vi "normalise_angle.vi"(10 "target -180 .. 180":dbl, 11 "current":dbl) -> (3 "travel_direction":dbl)   [LabVIEW 2017]
uses:
  <vilib>/Analysis/coordinate.llb/Angle Units.ctl
  <vilib>/Analysis/coordinate.llb/Absolute Angle Difference (scalar).vi
  <vilib>/Analysis/coordinate.llb/Wrap Angle (scalar).vi
  <vilib>/Analysis/coordinate.llb/Set Angle Unit.vi
  <vilib>/Analysis/NI_AAL_Angle.lvlib
panel:
  out "s? t:f":dbl
  out "absolute angle difference 2":dbl
  out "absolute angle difference":dbl
  out "current angle (-180..180)":dbl
  out "revolutions":dbl
  out "current angle (0... 359)":dbl
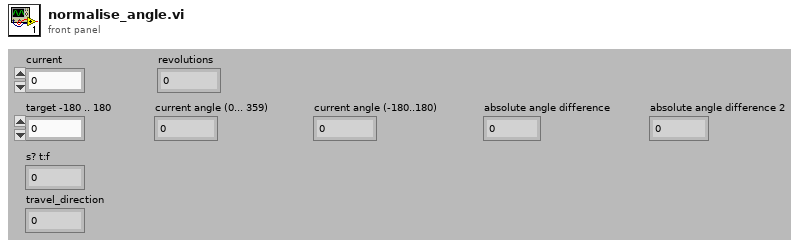
[diagram p1: front panel]
types:
  T1 = typedef "NI_AAL_Angle.lvlib/Angle Units.ctl" = i32
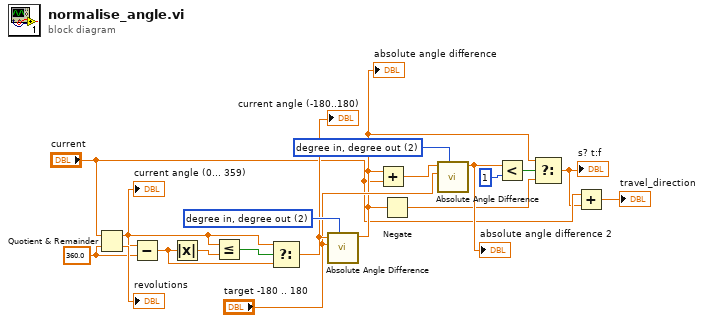
[diagram p0: block diagram]
diagram:
  w10 = T1 2 items=["radian in, radian out", "radian in, degree out", "degree in, degree out", "degree in, radian out"] ("angle units")
  w17 = 360.0 ("y")
  w19 = T1 2 items=["radian in, radian out", "radian in, degree out", "degree in, degree out", "degree in, radian out"] ("angle units")
  n1 = Quotient & Remainder(x="current", y=w17) -> (x-y*floor(x/y)=w14:dbl, floor(x/y)=→"revolutions":dbl)
  "current angle (0... 359)" <- w14
  n2 = Subtract(x=w14, y=w17) -> (x-y=w13:dbl)
  n3 = Absolute Value(x=w13) -> (abs(x)=w16:dbl)
  n4 = Less Or Equal?(x=w14, y=w16) -> (x <= y?=w15:bool)
  n5 = Select(t=w14, s=w15, f=w13) -> (s? t:f=w12:dbl)
  "current angle (-180..180)" <- w12
  n6 = call-poly <vilib>:"Absolute Angle Difference.vi"("angle units"=w19, "angle 2"="target -180 .. 180", "angle 1"=w12) -> ("absolute angle difference"=w4:dbl)  [unwired: 7 in, 1 out]
  "absolute angle difference" <- w4
  n7 = Add(x=w4, y="current") -> (x+y=w7:dbl)
  n8 = Negate(x=w4) -> (-x=w5:dbl)
  n9 = call-poly <vilib>:"Absolute Angle Difference.vi"("angle units"=w10, "angle 2"="target -180 .. 180", "angle 1"=w7) -> ("absolute angle difference"=w8:dbl)  [unwired: 7 in, 1 out]
  "absolute angle difference 2" <- w8
  n10 = Less?(x=w8, y=1) -> (x < y?=w6:bool)
  n11 = Select(t=w4, s=w6, f=w5) -> (s? t:f=w2:dbl)
  "s? t:f" <- w2
  n12 = Add(x="current", y=w2) -> (x+y=→"travel_direction":dbl)
